vi "Profile Auton - Distance.vi"(8 "error in (no error)":errorcluster, 10 "Time (s)":dbl format="%#_13g", 11 "Distance (ft)":dbl) -> (0 "error out":errorcluster)   [LabVIEW 2017]
uses:
  Robot Global Data.vi
  <vilib>/Rock Robotics/WPI/Utilities/WPI_GetSetVariantRefNum.vi
  <vilib>/Rock Robotics/Network Tables/NT Write Number.vi
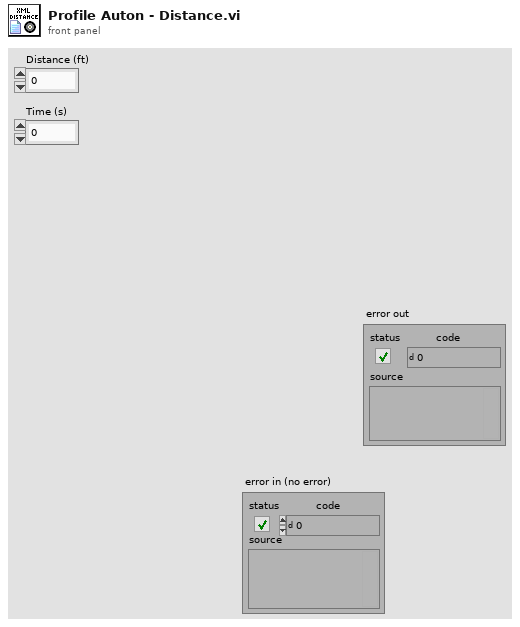
[diagram p1: front panel]
types:
  T1 = typedef "WPI_MotorControlDeviceRef.ctl" = cluster{"DeviceStatus":errorcluster, "Type":T2, "PWM":cluster{"PWM Channel":T3, "DeadBand":T4}, "CAN":cluster{"Device Number":u8, "SetOutput VI Ref":variant, "GetOutput VI Ref":variant, "Enable VI Ref":variant, "Disable VI Ref":variant, "Data":variant}, "Invert":bool, "DIO PWM":cluster{"PWM \"Enable\" Channel":T3, "DIOChannel":T5, "PWM Rate":dbl}}
  T2 = typedef "WPI_MotorControlType.ctl" = enum16{"PWM", "CAN", "DIO PWM"}
  T3 = typedef "FPGA_DIOPWMChannel.ctl" = enum8{"PWM 0", "PWM 1", "PWM 2", "PWM 3", "PWM 4", "PWM 5", "PWM 6", "PWM 7", "PWM 8", "PWM 9", "PWM MXP 0", "PWM MXP 1", "PWM MXP 2", "PWM MXP 3", "PWM MXP 4", "PWM MXP 5", "PWM MXP 6", "PWM MXP 7", "PWM MXP 8", "PWM MXP 9", "Invalid"}
  T4 = typedef "WPI_PWMDeadband.ctl" = cluster{"Name":string, "maxPositivePwm":i32, "minPositivePwm":i32, "centerPwm":i32, "maxNegativePwm":i32, "minNegativePwm":i32, "angularRange":u16}
  T5 = typedef "FPGA_DIOChannel.ctl" = enum8{"DIO 0", "DIO 1", "DIO 2", "DIO 3", "DIO 4", "DIO 5", "DIO 6", "DIO 7", "DIO 8", "DIO 9", "DIO MXP 0", "DIO MXP 1", "DIO MXP 2", "DIO MXP 3", "DIO MXP 4", "DIO MXP 5", "DIO MXP 6", "DIO MXP 7", "DIO MXP 8", "DIO MXP 9", "DIO MXP 10", "DIO MXP 11", "DIO MXP 12", "DIO MXP 13", "DIO MXP 14", "DIO MXP 15", "SPI Port CS1", "SPI Port CS2", "SPI Port CS3", "SPI Port MISO", "SPI Port MOSI", "Invalid"}
  T6 = typedef "WPI_RobotDriveDevRef.ctl" = cluster{"DevStatus":errorcluster, "Motors[]":T1[], "Square Inputs":bool, "Max Output":dbl}
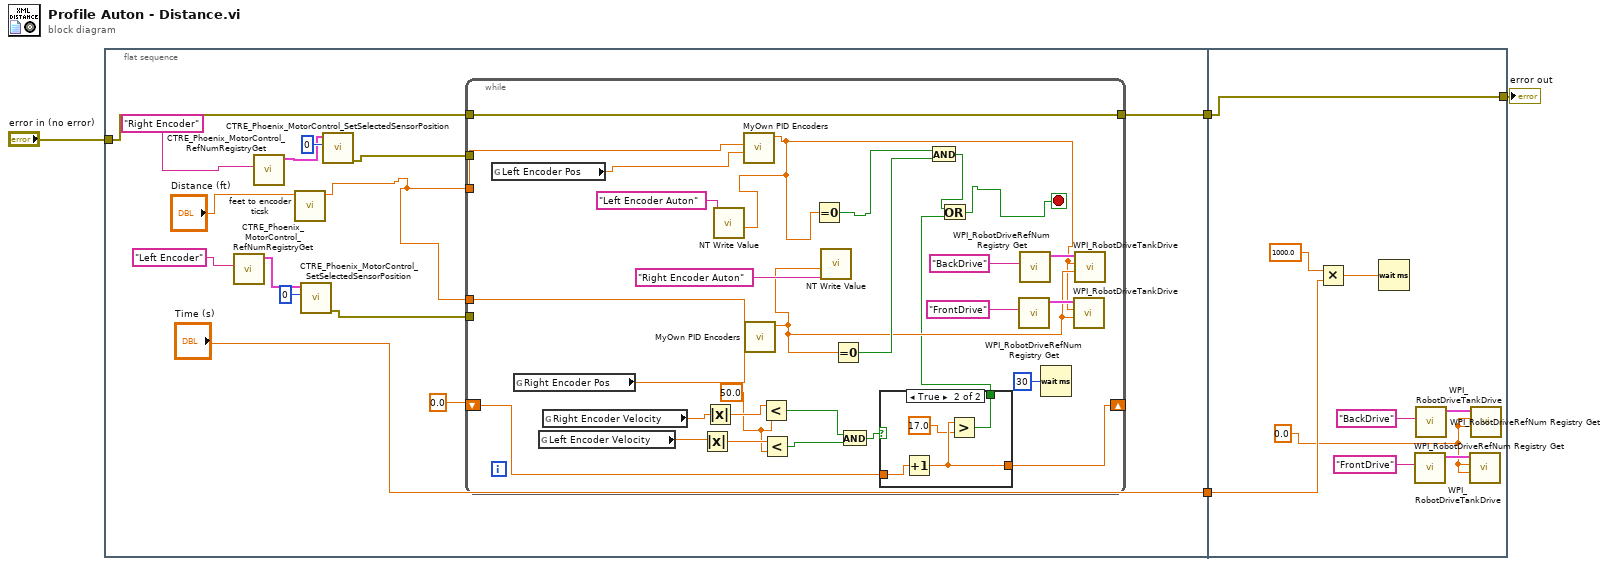
[diagram p0: block diagram]
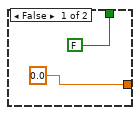
[diagram p2: hidden frame]
diagram:
  n1 = flat-sequence {
    tunnel: ["Time (s)"] -> w4
    tunnel: "error in (no error)" -> [w16]
    tunnel: [w15] -> w2
    tunnel: w4 -> [w61]
    tunnel: w2 -> [w59]
    tunnel: [w59] -> w1
    frame #0 {
      n2 = call <vilib>:"CTRE_Phoenix_MotorControl_RefNumRegistryGet.vi"("refnum name"="Left Encoder") -> ("PhoenixMotorControlDevRef"=w7:T1)  [unwired: 9 in, 1 out]
      n3 = call <vilib>:"CTRE_Phoenix_MotorControl_RefNumRegistryGet.vi"("refnum name"="Right Encoder") -> ("PhoenixMotorControlDevRef"=w8:T1)  [unwired: 9 in, 1 out]
      n4 = call "feet to encoder ticsk.vi"("Distance in feet wanted"="Distance (ft)") -> ("Encoder Ticks"=w14:dbl)  [unwired: 10 in]
      n5 = call <vilib>:"CTRE_Phoenix_MotorControl_SetSelectedSensorPosition.vi"("New Sensor Position"=0, "PhoenixMotorControlDevRef"=w7) -> ("error out"=w13:errorcluster)  [unwired: 8 in, 1 out]
      n6 = call <vilib>:"CTRE_Phoenix_MotorControl_SetSelectedSensorPosition.vi"("New Sensor Position"=0, "PhoenixMotorControlDevRef"=w8) -> ("error out"=w10:errorcluster)  [unwired: 8 in, 1 out]
      n7 = while {
        tunnel: w14 -> [w37]
        tunnel: w14 -> [w34]
        tunnel: w16 -> [w46]
        tunnel: [w46] -> w15
        tunnel: w13 -> [_]
        tunnel: w10 -> [_]
        shift-right: [w22] -> _
        shift-left: 0.0 -> [w23]
        stop <- w20 stop-if-true
        w27 = 50.0
        n8 = global read "Robot Global Data.vi" "Left Encoder Pos"() -> (w33:dbl)
        n9 = global read "Robot Global Data.vi" "Right Encoder Pos"() -> (w36:dbl)
        n10 = global read "Robot Global Data.vi" "Left Encoder Velocity"() -> (w31:dbl)
        n11 = global read "Robot Global Data.vi" "Right Encoder Velocity"() -> (w30:dbl)
        n12 = Absolute Value(x=w31) -> (abs(x)=w28:dbl)
        n13 = Absolute Value(x=w30) -> (abs(x)=w29:dbl)
        n14 = call "MyOwn PID Encoders.vi"("Current Input"=w33, "Wanted End"=w34) -> ("Output"=w32:dbl)  [unwired: 9 in]
        n15 = call-poly <vilib>:"NT Write Value.vi"("Numeric"=w32, "Name"="Left Encoder Auton") -> ()  [unwired: 9 in, 1 out]
        n16 = call "MyOwn PID Encoders.vi"("Current Input"=w36, "Wanted End"=w37) -> ("Output"=w35:dbl)  [unwired: 9 in]
        n17 = Less?(x=w29, y=w27) -> (x < y?=w25:bool)
        n18 = Less?(x=w28, y=w27) -> (x < y?=w24:bool)
        n19 = Equal To 0?(x=w32) -> (x = 0?=w43:bool)
        n20 = call-poly <vilib>:"NT Write Value.vi"("Numeric"=w35, "Name"="Right Encoder Auton") -> ()  [unwired: 9 in, 1 out]
        n21 = Equal To 0?(x=w35) -> (x = 0?=w42:bool)
        n22 = And(x=w25, y=w24) -> (x .and. y?=w26:bool)
        n23 = case shown="True" w26 {
          tunnel: w23 -> [_ w53]
          tunnel: [0.0 w52] -> w22
          tunnel: [FALSE w50] -> w19
          frame False {
          }
          frame True {
            n24 = Increment(x=w53) -> (x+1=w52:dbl)
            n25 = Greater?(x=w52, y=17.0) -> (0:w50:bool)
          }
        }
        n26 = And(x=w43, y=w42) -> (x .and. y?=w21:bool)
        n27 = Or(x=w21, y=w19) -> (x .or. y?=w20:bool)
        n28 = call <vilib>:"WPI_RobotDriveRefNum Registry Get.vi"("refnum name"="FrontDrive") -> ("RobotDriveDevRef"=w41:T6)  [unwired: 9 in, 1 out]
        n29 = call <vilib>:"WPI_RobotDriveRefNum Registry Get.vi"("refnum name"="BackDrive") -> ("RobotDriveDevRef"=w40:T6)  [unwired: 9 in, 1 out]
        n30 = Wait (ms)(milliseconds to wait=u32 30) -> ()  [unwired: 1 out]
        n31 = call <vilib>:"WPI_RobotDriveTankDrive.vi"("Right axis value"=w35, "Left axis value"=w32, "RobotDriveDevRef"=w41) -> ()  [unwired: 6 in, 3 out]
        n32 = call <vilib>:"WPI_RobotDriveTankDrive.vi"("Right axis value"=w35, "Left axis value"=w32, "RobotDriveDevRef"=w40) -> ()  [unwired: 6 in, 3 out]
      }
    }
    frame #1 {
      w54 = 0.0
      n33 = Multiply(x=1000.0, y=w61) -> (x*y=w62:dbl)
      n34 = Wait (ms)(milliseconds to wait=w62) -> ()  [unwired: 1 out]
      n35 = call <vilib>:"WPI_RobotDriveRefNum Registry Get.vi"("refnum name"="FrontDrive") -> ("RobotDriveDevRef"=w55:T6)  [unwired: 9 in, 1 out]
      n36 = call <vilib>:"WPI_RobotDriveRefNum Registry Get.vi"("refnum name"="BackDrive") -> ("RobotDriveDevRef"=w56:T6)  [unwired: 9 in, 1 out]
      n37 = call <vilib>:"WPI_RobotDriveTankDrive.vi"("Right axis value"=w54, "Left axis value"=w54, "RobotDriveDevRef"=w55) -> ()  [unwired: 6 in, 3 out]
      n38 = call <vilib>:"WPI_RobotDriveTankDrive.vi"("Right axis value"=w54, "Left axis value"=w54, "RobotDriveDevRef"=w56) -> ()  [unwired: 6 in, 3 out]
    }
  }
  "error out" <- w1
